vi "Main_with_Timeout.vi"() -> ()   [LabVIEW 2020]
uses:
  #typedef_TeacherDataBase.ctl
  #typedes_ActionsTime.ctl
  #typedef_action.ctl
panel:
  out "English":string
  out "Polish":string
  in  "Exit":bool
  in  "Stop":bool
  in  "Start Test":bool
  in  "Start Learning":bool
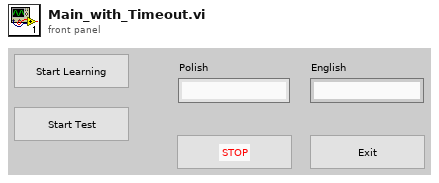
[diagram p1: front panel]
types:
  T1 = typedef "#typedef_action.ctl" = enum16{"Initialize", "Idle", "Start Learning", "Learning_PolishWord", "Learning_EnglishWord", "Wait", "Start Test", "Test_EnterWord", "Test_Check", "Stop", "Exit"}
  T2 = typedef "#typedef_TeacherDataBase.ctl" = cluster{"English":path, "Polish":path, "Cluster":T3, "Current index ":dbl, "Current English Word":string}
  T3 = typedef "#typedes_ActionsTime.ctl" = cluster{"Start Learning":dbl, "Start Learning Polish":dbl, "Start Learning English":dbl}
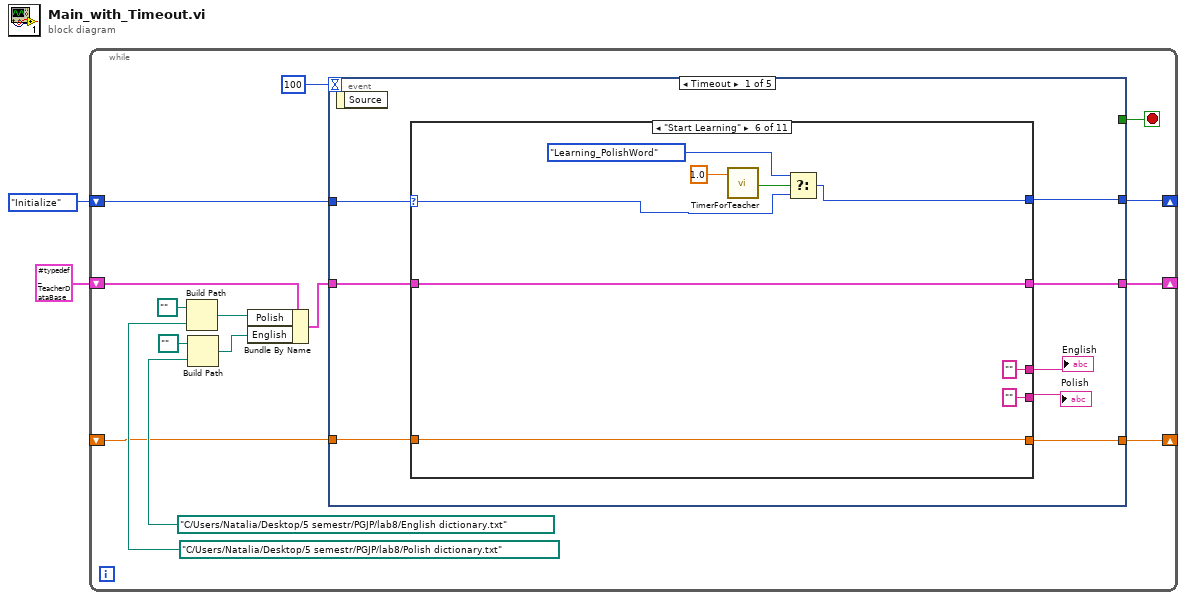
[diagram p0: block diagram]
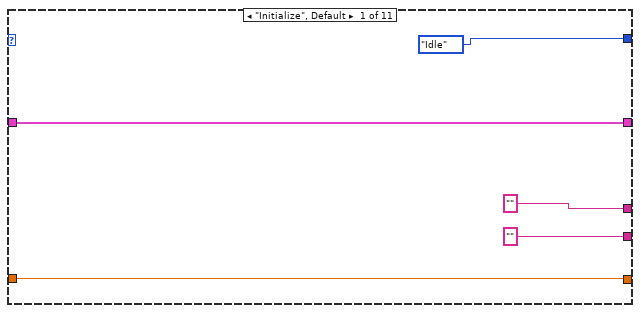
[diagram p2: hidden frame]
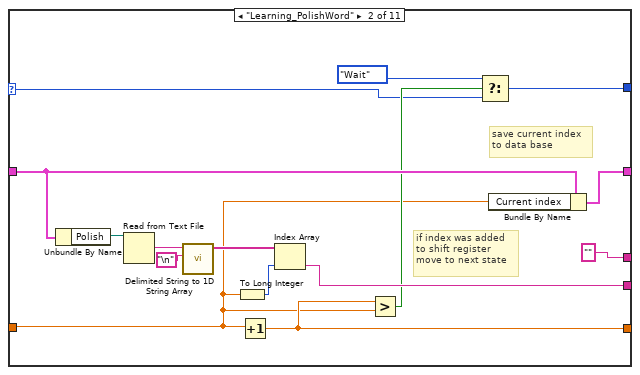
[diagram p3: hidden frame]
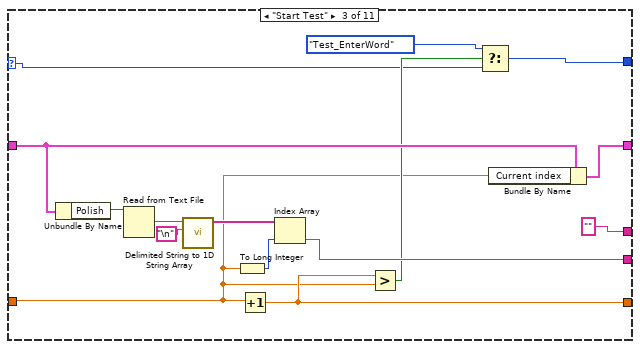
[diagram p4: hidden frame]
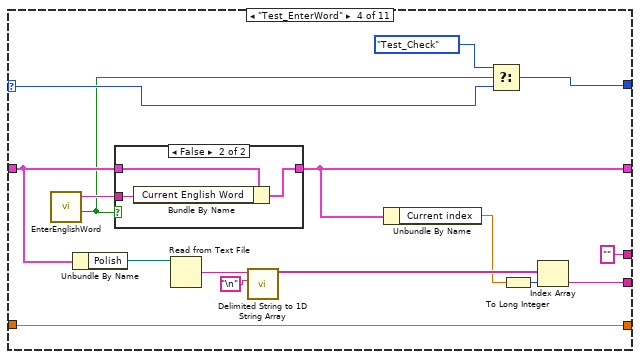
[diagram p5: hidden frame]
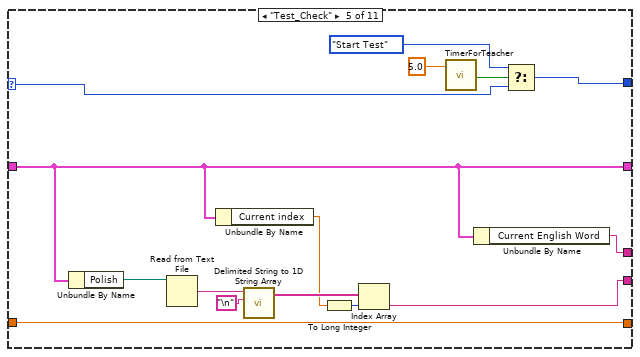
[diagram p7: hidden frame]
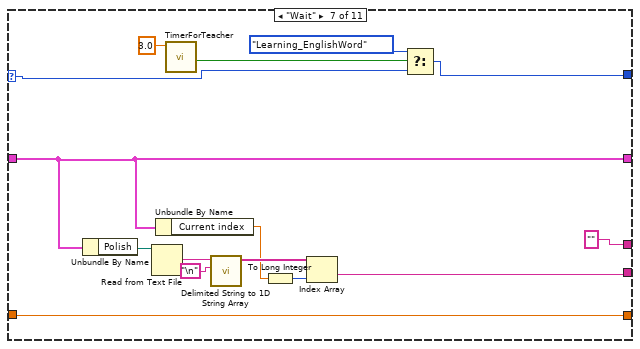
[diagram p8: hidden frame]
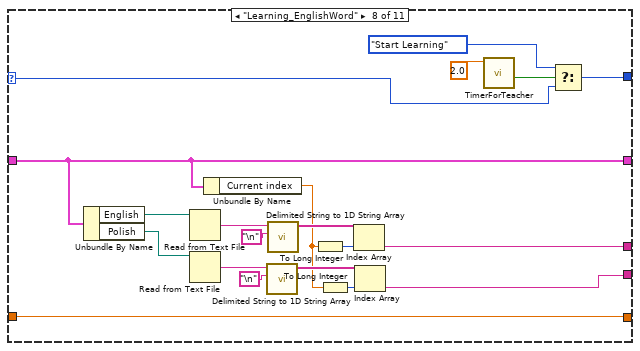
[diagram p9: hidden frame]
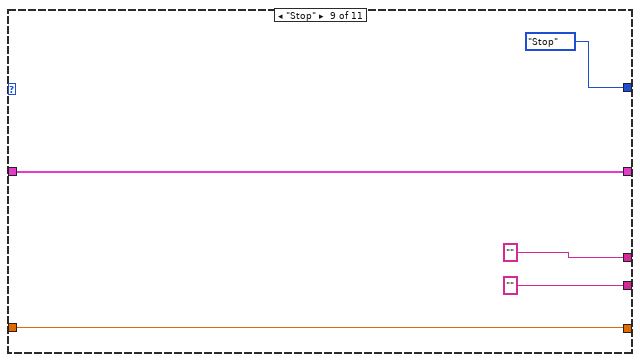
[diagram p10: hidden frame]
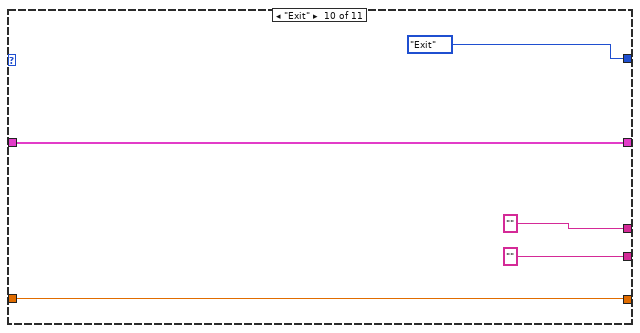
[diagram p11: hidden frame]
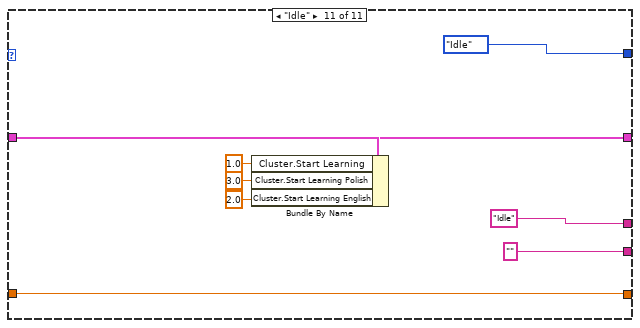
[diagram p12: hidden frame]
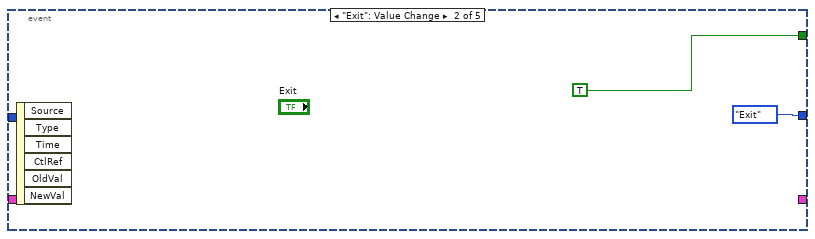
[diagram p13: hidden frame]
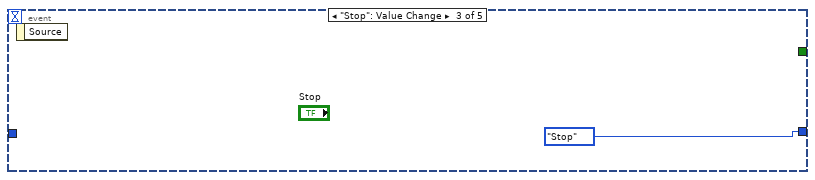
[diagram p14: hidden frame]
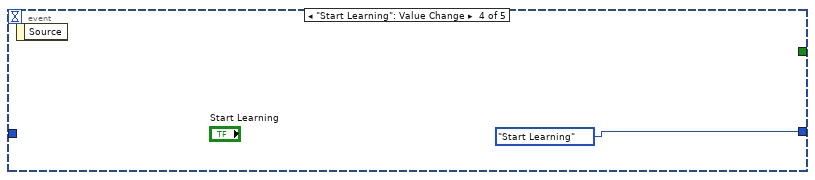
[diagram p15: hidden frame]
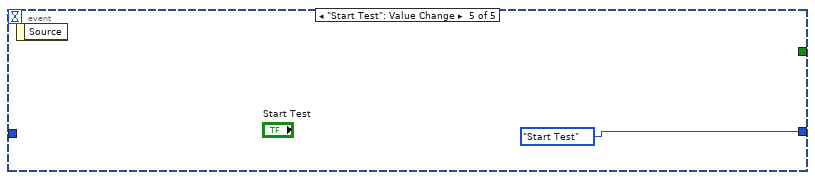
[diagram p16: hidden frame]
diagram:
  n1 = while {
    shift-right: [w15] -> _
    shift-left: T2 {"English"=path "", "Polish"=path "", "Cluster"={"Start Learning"=0.0, "Start Learning Polish"=0.0, "Start Learning English"=0.0}, "Current index "=0.0, "Current English Word"=""} ("Data Base") -> [w8]
    shift-right: [w5] -> _
    shift-left: _ -> [w6]
    shift-right: [w3] -> _
    shift-left: #typedef_action."Initialize" ("Action") -> [w4]
    stop <- w17 stop-if-true
    n2 = Build Path(base path=path "", name or relative path=path "C:/Users/Natalia/Desktop/5 semestr/PGJP/lab8/Polish dictionary.txt") -> (appended path=w13:path)
    n3 = Build Path(base path=path "", name or relative path=path "C:/Users/Natalia/Desktop/5 semestr/PGJP/lab8/English dictionary.txt") -> (appended path=w12:path)
    n4 = Bundle By Name(cluster=w8, "Polish"=w13, "English"=w12) -> (w7:T2)
    n5 = event shown="[0] Timeout" {
      selector: _ -> [_ _ _ _ _]
      dyn-events: _ -> [_ _ _ _ _]
      timeout: 100 -> [_ _ _ _ _]
      tunnel: [_ TRUE _ _ _] -> w17
      tunnel: [w25 _ _ _ _] -> w15
      tunnel: w7 -> [w24 _ _ _ _]
      tunnel: w6 -> [w21 _ _ _ _]
      tunnel: [w20 _ _ _ _] -> w5
      tunnel: w4 -> [w19 _ _ _ _]
      tunnel: [w18 #typedef_action."Exit" ("Action") #typedef_action."Stop" ("Action") #typedef_action."Start Learning" ("Action") #typedef_action."Start Test" ("Action")] -> w3
      event Timeout {
        n6 = event-data() -> ()  [unwired: 1 in, 1 out]
        n7 = case shown="\"Start Learning\"" w19 {
          selector: w19 -> [_ w32 w47 w66 w83 w99 w107 w120 _ _ _]
          tunnel: [w28 w37 w52 w62 w82 w100 w110 w130 w142 w149 w155] -> w25
          tunnel: w24 -> [w28 w38 w53 w64 w82 w100 w110 w130 w142 w149 w156]
          tunnel: ["" ("String") "" ("String") "" ("String") "" ("String") w81 "" ("String") "" ("String") w122 "" ("String") "" ("String") "Idle" ("String")] -> w23
          tunnel: ["" w40 w55 w70 w88 "" ("String") w113 w131 "" "" ""] -> w22
          tunnel: w21 -> [w27 w34 w49 w69 w95 w104 w112 w132 w141 w146 w151]
          tunnel: [w27 w39 w54 w69 w95 w104 w112 w132 w141 w146 w151] -> w20
          tunnel: [#typedef_action."Idle" ("Action") w31 w46 w67 w84 w98 w105 w121 #typedef_action."Stop" ("Action") #typedef_action."Exit" ("Action") #typedef_action."Idle" ("Action")] -> w18
          frame "Initialize", Default {
          }
          frame "Learning_PolishWord" {
            # "save current index \nto data base"
            # "if index was added \nto shift register\nmove to next state"
            n8 = Unbundle By Name(w38) -> ("Polish"=w44:path)
            n9 = Read from Text File(file (use dialog)=w44) -> (text=w43:string)  [unwired: 3 in, 3 out]
            n10 = call <vilib>:"Delimited String to 1D String Array.vi"("delimiter"="\n", "delimited string"=w43) -> ("string array"=w41:string[])  [unwired: 9 in]
            n11 = To Long Integer(number=w34) -> (32bit integer=w35:i32)
            n12 = Increment(x=w34) -> (x+1=w39:dbl)
            n13 = Index Array(array=w41, index=w35) -> (element=w40:string)
            n14 = Greater?(x=w39, y=w34) -> (0:w36:bool)
            n15 = Select(t=#typedef_action."Wait" ("Action"), s=w36, f=w32) -> (s? t:f=w31:T1)
            n16 = Bundle By Name(cluster=w38, "Current index"=w34) -> (w37:T2)
          }
          frame "Start Test" {
            n17 = Unbundle By Name(w53) -> ("Polish"=w59:path)
            n18 = Read from Text File(file (use dialog)=w59) -> (text=w58:string)  [unwired: 3 in, 3 out]
            n19 = call <vilib>:"Delimited String to 1D String Array.vi"("delimiter"="\n", "delimited string"=w58) -> ("string array"=w56:string[])  [unwired: 9 in]
            n20 = To Long Integer(number=w49) -> (32bit integer=w50:i32)
            n21 = Increment(x=w49) -> (x+1=w54:dbl)
            n22 = Index Array(array=w56, index=w50) -> (element=w55:string)
            n23 = Greater?(x=w54, y=w49) -> (0:w51:bool)
            n24 = Select(t=#typedef_action."Test_EnterWord" ("Action"), s=w51, f=w47) -> (s? t:f=w46:T1)
            n25 = Bundle By Name(cluster=w53, "Current index"=w49) -> (w52:T2)
          }
          frame "Test_EnterWord" {
            n26 = call "EnterEnglishWord.vi"() -> ("Cancelled"=w63:bool, "English"=w65:string)  [unwired: 9 in, 1 out]
            n27 = Unbundle By Name(w64) -> ("Polish"=w76:path)
            n28 = case shown="False" w63 {
              tunnel: w65 -> [_ w80]
              tunnel: w64 -> [w77 w79]
              tunnel: [w77 w78] -> w62
              frame True {
              }
              frame False {
                n29 = Bundle By Name(cluster=w79, "Current English Word"=w80) -> (w78:T2)
              }
            }
            n30 = Read from Text File(file (use dialog)=w76) -> (text=w75:string)  [unwired: 3 in, 3 out]
            n31 = call <vilib>:"Delimited String to 1D String Array.vi"("delimiter"="\n", "delimited string"=w75) -> ("string array"=w73:string[])  [unwired: 9 in]
            n32 = Unbundle By Name(w62) -> ("Current index"=w72:dbl)
            n33 = Select(t=#typedef_action."Test_Check" ("Action"), s=w63, f=w66) -> (s? t:f=w67:T1)
            n34 = To Long Integer(number=w72) -> (32bit integer=w71:i32)
            n35 = Index Array(array=w73, index=w71) -> (element=w70:string)
          }
          frame "Test_Check" {
            n36 = Unbundle By Name(w82) -> ("Polish"=w94:path)
            n37 = Read from Text File(file (use dialog)=w94) -> (text=w93:string)  [unwired: 3 in, 3 out]
            n38 = Unbundle By Name(w82) -> ("Current index"=w89:dbl)
            n39 = call <vilib>:"Delimited String to 1D String Array.vi"("delimiter"="\n", "delimited string"=w93) -> ("string array"=w91:string[])  [unwired: 9 in]
            n40 = To Long Integer(number=w89) -> (32bit integer=w90:i32)
            n41 = Index Array(array=w91, index=w90) -> (element=w88:string)
            n42 = call "TimerForTeacher.vi"("Time to Elapse (2s)"=5.0) -> ("Time Elapsed?"=w87:bool)  [unwired: 8 in, 2 out]
            n43 = Unbundle By Name(w82) -> ("Current English Word"=w81:string)
            n44 = Select(t=#typedef_action."Start Test" ("Action"), s=w87, f=w83) -> (s? t:f=w84:T1)
          }
          frame "Start Learning" {
            n45 = call "TimerForTeacher.vi"("Time to Elapse (2s)"=1.0) -> ("Time Elapsed?"=w103:bool)  [unwired: 8 in, 2 out]
            n46 = Select(t=#typedef_action."Learning_PolishWord" ("Action"), s=w103, f=w99) -> (s? t:f=w98:T1)
          }
          frame "Wait" {
            n47 = Unbundle By Name(w110) -> ("Polish"=w117:path)
            n48 = Read from Text File(file (use dialog)=w117) -> (text=w116:string)  [unwired: 3 in, 3 out]
            n49 = Unbundle By Name(w110) -> ("Current index"=w109:dbl)
            n50 = call "TimerForTeacher.vi"("Time to Elapse (2s)"=3.0) -> ("Time Elapsed?"=w111:bool)  [unwired: 8 in, 2 out]
            n51 = call <vilib>:"Delimited String to 1D String Array.vi"("delimiter"="\n", "delimited string"=w116) -> ("string array"=w114:string[])  [unwired: 9 in]
            n52 = To Long Integer(number=w109) -> (32bit integer=w108:i32)
            n53 = Index Array(array=w114, index=w108) -> (element=w113:string)
            n54 = Select(t=#typedef_action."Learning_EnglishWord", s=w111, f=w107) -> (s? t:f=w105:T1)
          }
          frame "Learning_EnglishWord" {
            n55 = Unbundle By Name(w130) -> ("English"=w126:path, "Polish"=w136:path)
            n56 = Read from Text File(file (use dialog)=w126) -> (text=w129:string)  [unwired: 3 in, 3 out]
            n57 = Read from Text File(file (use dialog)=w136) -> (text=w135:string)  [unwired: 3 in, 3 out]
            n58 = Unbundle By Name(w130) -> ("Current index"=w124:dbl)
            n59 = call <vilib>:"Delimited String to 1D String Array.vi"("delimiter"="\n", "delimited string"=w135) -> ("string array"=w133:string[])  [unwired: 9 in]
            n60 = call <vilib>:"Delimited String to 1D String Array.vi"("delimiter"="\n", "delimited string"=w129) -> ("string array"=w127:string[])  [unwired: 9 in]
            n61 = To Long Integer(number=w124) -> (32bit integer=w125:i32)
            n62 = To Long Integer(number=w124) -> (32bit integer=w123:i32)
            n63 = Index Array(array=w127, index=w125) -> (element=w122:string)
            n64 = Index Array(array=w133, index=w123) -> (element=w131:string)
            n65 = call "TimerForTeacher.vi"("Time to Elapse (2s)"=2.0) -> ("Time Elapsed?"=w139:bool)  [unwired: 8 in, 2 out]
            n66 = Select(t=#typedef_action."Start Learning" ("Action"), s=w139, f=w120) -> (s? t:f=w121:T1)
          }
          frame "Stop" {
          }
          frame "Exit" {
          }
          frame "Idle" {
            n67 = Bundle By Name(cluster=w156, "Cluster.Start Learning"=1.0, "Cluster.Start Learning Polish"=3.0, "Cluster.Start Learning English"=2.0) -> (w155:T2)
          }
        }
        "Polish" <- w22
        "English" <- w23
      }
      event "Exit": Value Change {
        n68 = event-data() -> ()  [unwired: 1 in, 6 out]
      }
      event "Stop": Value Change {
        n69 = event-data() -> ()  [unwired: 1 in, 1 out]
      }
      event "Start Learning": Value Change {
        n70 = event-data() -> ()  [unwired: 1 in, 1 out]
      }
      event "Start Test": Value Change {
        n71 = event-data() -> ()  [unwired: 1 in, 1 out]
      }
    }
  }
